vi "VA CoAP - Insert String into JSON.vi"(8 "error in (no error)":errorcluster, 9 "Element value":T1, 10 "Element name":string, 11 "JSON Value in":refnum<class "JSON Value.lvclass">) -> (0 "error out":errorcluster, 3 "JSON Value out":refnum<class "JSON Value.lvclass">)   [LabVIEW 2020]
uses:
  data types/MEEB Dock CoAP - Command.ctl
  <vilib>/addons/JSON API/JSON Value/JSON Value.lvclass
  <vilib>/addons/JSON API/JSON Scalar/JSON Scalar.lvclass/JSON Scalar.ctl
  <vilib>/addons/JSON API/JSON Scalar/Quote and Escape JSON string.vi
  <vilib>/addons/JSON API/JSON Scalar/JSON Scalar.lvclass
  c:/Program Files (x86)/National Instruments/LabVIEW 2020/vi.lib/addons/JSON API/JSON Value/JSON Value.lvclass
  <vilib>/addons/JSON API/JSON Value/Set Item by name array.vi
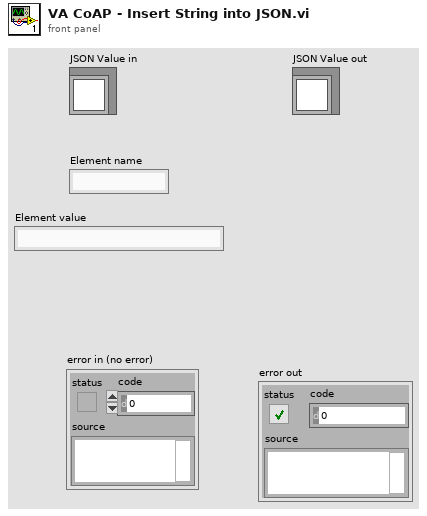
[diagram p1: front panel]
types:
  T1 = typedef "MEEB Dock CoAP - Command.ctl" = string
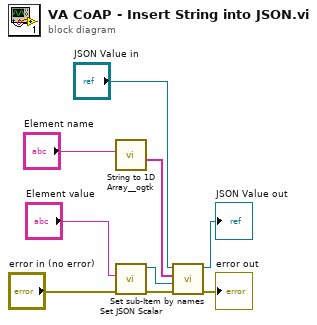
[diagram p0: block diagram]
diagram:
  n1 = call <userlib>:"String to 1D Array__ogtk.vi"("string"="Element name") -> ("Array of Strings"=w8:string[])  [unwired: 10 in]
  n2 = call <vilib>:"Set JSON Scalar.vi"("error in (no error)"="error in (no error)", "LabVIEW Text"="Element value") -> ("error out"=w5:errorcluster, "JSON Scalar out"=w9:refnum<class "JSON Scalar.lvclass">)  [unwired: 8 in]
  n3 = call <vilib>:"Set sub-Item by names.vi"("error in (no error)"=w5, "Value"=w9, "Name Array"=w8, "JSON Value In"="JSON Value in") -> ("error out"=→"error out":errorcluster, "JSON Value Out"=→"JSON Value out":refnum<class "JSON Value.lvclass">)  [unwired: 5 in, 1 out]
